vi "TCP Server Create.vi"(6 "Additional Data":variant, 7 "net address (0: Listen on All Adaptors)":u32, 8 "error in (no error)":errorcluster, 9 "max connections (0: no limit)":u32, 10 "port":u16, 11 "Connection Handler Call-Back VI RefNum":T1) -> (0 "error out":errorcluster, 3 "TCP Server":refnum<class "JKI TCP Server.lvclass">)   [LabVIEW 2020, in "JKI TCP Server.lvclass"]
uses:
  JKI TCP Server.lvclass
  _Data Structures/TCP Server Data.ctl
  _Data Structures/TCP Server Listener Info Cluster.ctl
  _Data Structures/TCP Server Connection Info Cluster.ctl
  _Data Structures/TCP Server Handler RefNum.ctl
  _Processes/TCP Server Listener Process.vi
  JKI TCP Server.lvclass/JKI TCP Server.ctl
panel:
  in  "Data in":T2
  # "Copyright © 2004-2008 JKI. All rights reserved.\n\nAuthor: Jim Kring [jim.kring@jameskring.com]\n\nThis library is provided \"AS IS\" ,WITHOUT WARRANTIES OR \nCONDITIONS OF ANY KIND, either express or implied.\n\nJames Kring, Inc. -- http://www.jameskring.com"
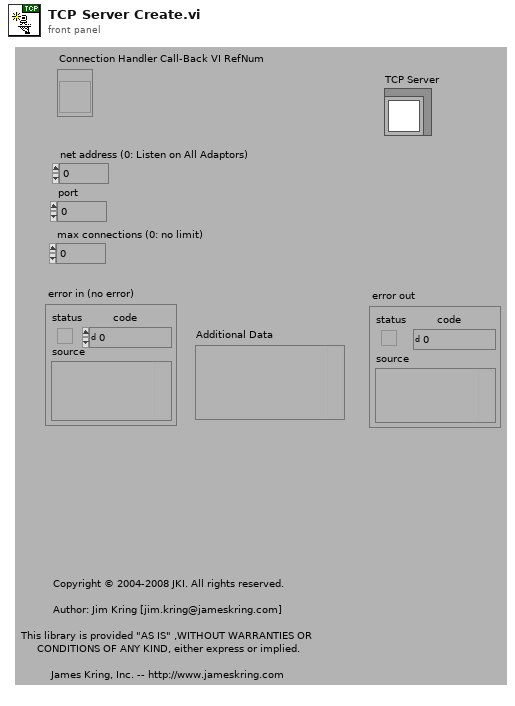
[diagram p1: front panel]
types:
  T1 = typedef "JKI TCP Server.lvclass/TCP Server Handler RefNum.ctl" = refnum<vi>
  T2 = typedef "JKI TCP Server.lvclass/TCP Server Data.ctl" = cluster{"Listener Info":T3, "Connection Process VI RefNums":refnum<vi>[], "dup connection IDs (for quick search)":refnum<k5>[], "Connections":T4[], "Connection Handler VI Path":path, "Handler Is Reentrant?":bool, "TCP Handler Instance RefNums":T1[], "TCP Handler VI RefNum":T1, "No. Connections":u32, "Max Connections":u32, "server start time":u32, "Additional Data":variant}
  T3 = typedef "JKI TCP Server.lvclass/TCP Server Listener Info Cluster.ctl" = cluster{"listener ID":refnum<k5>, "net address":u32, "port":u16, "Listener Process VI Refnum":refnum<vi>}
  T4 = typedef "JKI TCP Server.lvclass/TCP Server Connection Info Cluster.ctl" = cluster{"connection ID":refnum<k5>, "Remote Address":string, "remote port":u16, "connection start time":u32}
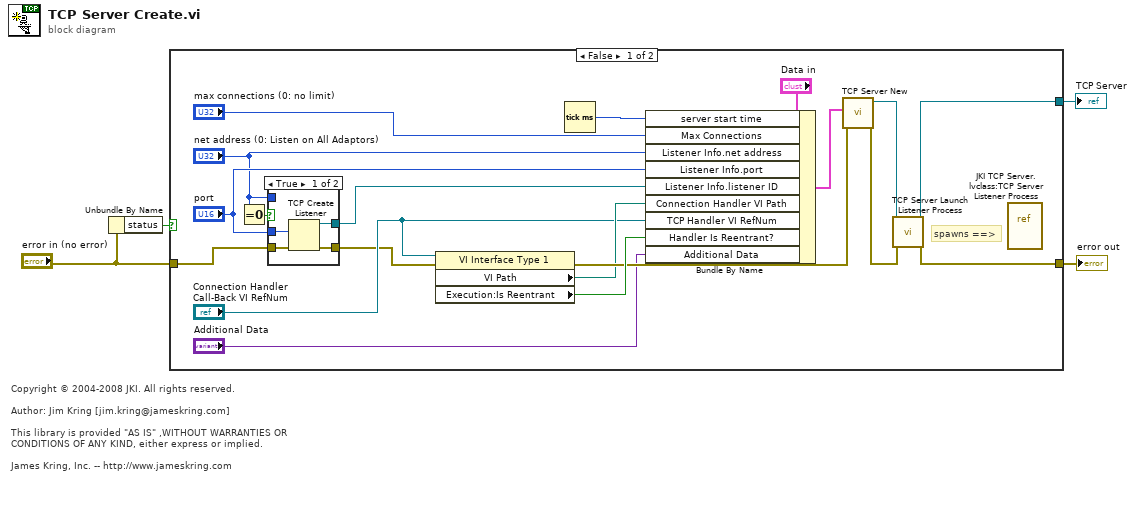
[diagram p0: block diagram]
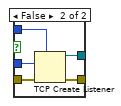
[diagram p2: hidden frame]
diagram:
  # "Copyright © 2004-2008 JKI. All rights reserved.\n\nAuthor: Jim Kring [jim.kring@jameskring.com]\n\nThis library is provided \"AS IS\" ,WITHOUT WARRANTIES OR \nCONDITIONS OF ANY KIND, either express or implied.\n\nJames Kring, Inc. -- http://www.jameskring.com"
  n1 = Unbundle By Name("error in (no error)") -> ("status"=w4:bool)
  n2 = case shown="False" w4 {
    tunnel: "error in (no error)" -> [w19 w33]
    tunnel: [w17 w33] -> w2
    tunnel: [w15 _] -> w1
    frame False {
      # "spawns ==>"
      n3 = Equal To 0?(x="net address (0: Listen on All Adaptors)") -> (x = 0?=w14:bool)
      n4 = case shown="True" w14 {
        tunnel: "port" -> [w27 w32]
        tunnel: [w26 w31] -> w20
        tunnel: w19 -> [w25 w30]
        tunnel: [w24 w29] -> w6
        tunnel: "net address (0: Listen on All Adaptors)" -> [_ w28]
        frame True {
          n5 = TCP Create Listener(8:w25, 10:w27) -> (0:w24:errorcluster, 3:w26:refnum<k5>)  [unwired: 3 in, 1 out]
        }
        frame False {
          n6 = TCP Create Listener(7:w28, 8:w30, 10:w32) -> (0:w29:errorcluster, 3:w31:refnum<k5>)  [unwired: 2 in, 1 out]
        }
      }
      n7 = property class="VI Interface Type 1"(reference="Connection Handler Call-Back VI RefNum", error in=w6) -> (error out=w11:errorcluster, "VI Path"=w8:path, "Execution:Is Reentrant"=w12:bool)  [unwired: 1 out]
      n8 = Tick Count (ms)() -> (millisecond timer value=w9:u32)
      n9 = Bundle By Name(cluster="Data in", "server start time"=w9, "Max Connections"="max connections (0: no limit)", "Listener Info.net address"="net address (0: Listen on All Adaptors)", "Listener Info.port"="port", "Listener Info.listener ID"=w20, "Connection Handler VI Path"=w8, "TCP Handler VI RefNum"="Connection Handler Call-Back VI RefNum", "Handler Is Reentrant?"=w12, "Additional Data"="Additional Data") -> (w23:T2)
      n10 = call "TCP Server New.vi"("error in (no error)"=w11, "Data in"=w23) -> ("error out"=w18:errorcluster, "TCP Server RefNum"=w16:refnum<class "JKI TCP Server.lvclass">)  [unwired: 8 in]
      n11 = call "TCP Server Launch Listener Process.vi"("error out"=w18, "RefNum"=w16) -> ("error"=w17:errorcluster, "dup RefNum"=w15:refnum<class "JKI TCP Server.lvclass">)  [unwired: 8 in]
      n12 = vi-ref "JKI TCP Server.lvclass:TCP Server Listener Process.vi"() -> ()  [unwired: 1 out]
    }
    frame True {
    }
  }
  "error out" <- w2
  "TCP Server" <- w1
